vi "SetUnit.vi"(8 "error in":errorcluster, 10 "Unit":T1, 11 "Measure in":refnum<class "Measure.lvclass">) -> (0 "error out":errorcluster, 3 "Measure out":refnum<class "Measure.lvclass">)   [LabVIEW 2021, in "ProligentXMLGenerator.lvlib" / "Measure.lvclass"]
doc: "Defines the name of the unit of the measure value (Ex: kilometer). When a unit symbol is provided, the unit name becomes required.\nDefines the symbol of the unit for the measure value (ex: km). When a unit name is provided, the unit symbol becomes required.\n\nUnit Name vaule is restricted to 30 characters and Unit Symbol is restricted to 20 characters."
uses:
  Measure.lvclass
  Measure.lvclass/Measure.ctl
  Base/Attribute/Attribute.lvclass
  Base/NonEmptyString_20/NonEmptyString_20.lvclass
  Base/NonEmptyString_30/NonEmptyString_30.lvclass
  C:/Projects/proligent-xml-generator-labview/src/ProligentXMLGenerator/Base/NonEmptyString/NonEmptyString.lvclass
  C:/Projects/proligent-xml-generator-labview/src/ProligentXMLGenerator/Base/String/String.lvclass
  C:/Projects/proligent-xml-generator-labview/src/ProligentXMLGenerator/Base/Attribute/Attribute.lvclass
  C:/Projects/proligent-xml-generator-labview/src/ProligentXMLGenerator/Base/NonEmptyString_30/NonEmptyString_30.lvclass
  Unit.ctl
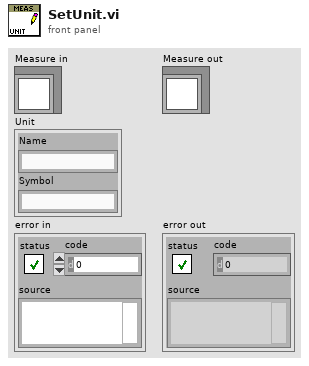
[diagram p1: front panel]
types:
  T1 = typedef "ProligentXMLGenerator.lvlib/Measure.lvclass/Unit.ctl" = cluster{"Name":string, "Symbol":string}
  T2 = typedef "ProligentXMLGenerator.lvlib/Measure.lvclass/Data.ctl" = cluster{"Name":string, "Type":refnum<class "MeasureKind.lvclass">, "Precision":refnum<class "UnsignedByte.lvclass">, "Limit":refnum<class "MeasureLimit.lvclass">, "Characteristics":refnum<class "Characteristic.lvclass">[], "FailureReferences":refnum<class "FailureReference.lvclass">[], "CustomData":refnum<class "CustomData.lvclass">, "MeasureId":refnum<class "Guid.lvclass">, "MeasureTime":refnum<class "DateTime.lvclass">, "Comments":refnum<class "NonNullableString_TruncateAt_255.lvclass">, "Unit":refnum<class "NonEmptyString_30.lvclass">, "Symbol":refnum<class "NonEmptyString_20.lvclass">, "MeasureExecutionStatus":refnum<class "ExecutionStatus.lvclass">}
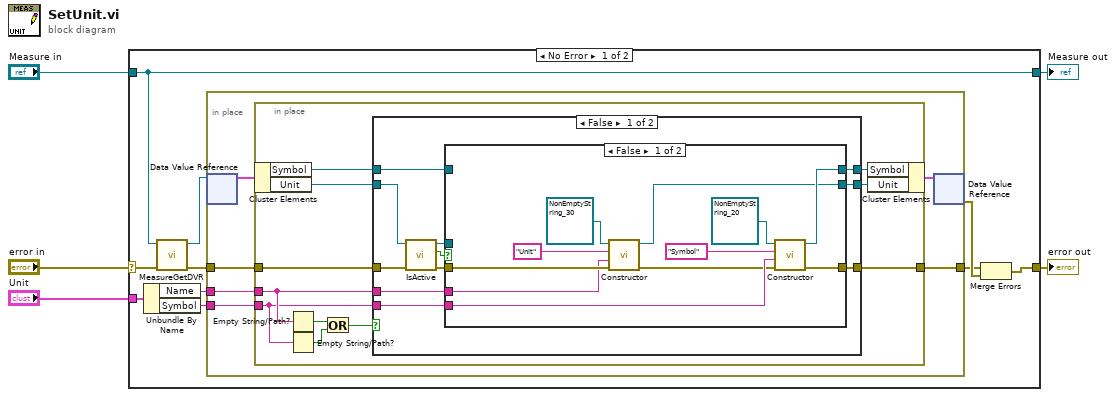
[diagram p0: block diagram]
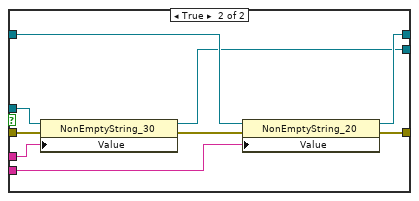
[diagram p2: hidden frame]
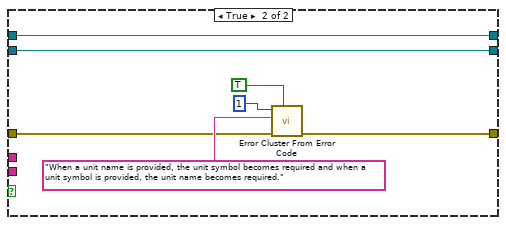
[diagram p3: hidden frame]
diagram:
  n1 = case shown="No Error" "error in" {
    selector: "error in" -> [w13 w71]
    tunnel: "Measure in" -> [w8 w72]
    tunnel: [w10 w71] -> w3
    tunnel: "Unit" -> [w9 _]
    tunnel: [w8 w72] -> w1
    frame No Error {
      n2 = Unbundle By Name(w9) -> ("Name"=w7:string, "Symbol"=w6:string)
      n3 = call "MeasureGetDVR.vi"("error in"=w13, "Measure"=w8) -> ("error out"=w12:errorcluster, "DVRReference"=w14:refnum<data-value>)  [unwired: 8 in]
      n4 = in-place "In Place Element Structure" {
        in-place-border: w12 -> [w21]
        in-place-border: [w20] -> w11
        in-place-border: w7 -> [w19]
        in-place-border: w6 -> [w16]
        n5 = in-place-dvr #1(w14) -> (w18:T2)  [unwired: 1 out]
        n6 = in-place "In Place Element Structure" {
          in-place-border: w21 -> [w25]
          in-place-border: [w32] -> w20
          in-place-border: w19 -> [w24]
          in-place-border: w16 -> [w23]
          n7 = in-place-cluster #2(w18) -> ("Symbol"=w31:refnum<class "NonEmptyString_20.lvclass">, "Unit"=w26:refnum<class "NonEmptyString_30.lvclass">)
          n8 = Empty String/Path?(string/path=w24) -> (empty?=w29:bool)
          n9 = Empty String/Path?(string/path=w23) -> (empty?=w28:bool)
          n10 = Or(x=w29, y=w28) -> (x .or. y?=w22:bool)
          n11 = case shown="False" w22 {
            tunnel: [w43 w68] -> w32
            tunnel: w31 -> [w42 w67]
            tunnel: [w41 w67] -> w30
            tunnel: [w40 w66] -> w27
            tunnel: w26 -> [w39 w66]
            tunnel: w25 -> [w38 w64]
            tunnel: w24 -> [w34 _]
            tunnel: w23 -> [w33 _]
            frame False {
              n12 = call "IsActive.vi"("error in"=w38, "Attribute in"=w39) -> ("error out"=w37:errorcluster, "IsActive"=w36:bool, "Attribute in"=w35:refnum<class "NonEmptyString_30.lvclass">)  [unwired: 7 in]
              n13 = case shown="False" w36 {
                tunnel: w37 -> [w47 w56]
                tunnel: [w52 w63] -> w43
                tunnel: w42 -> [_ w62]
                tunnel: [w54 w61] -> w41
                tunnel: [w45 w60] -> w40
                tunnel: w35 -> [_ w59]
                tunnel: w34 -> [w44 w58]
                tunnel: w33 -> [w53 w57]
                frame False {
                  n14 = call-dynamic "Constructor.vi"("error in"=w47, "Value"=w44, "Name"="Unit", "String in"=refnum<class "NonEmptyString_30.lvclass"> refnum ("ProligentResultProcessor:NonEmptyString_30")) -> ("error out"=w46:errorcluster, "String out"=w45:refnum<class "NonEmptyString_30.lvclass">)  [unwired: 6 in]
                  n15 = call-dynamic "Constructor.vi"("error in"=w46, "Value"=w53, "Name"="Symbol", "String in"=refnum<class "NonEmptyString_20.lvclass"> refnum ("ProligentResultProcessor:NonEmptyString_20")) -> ("error out"=w52:errorcluster, "String out"=w54:refnum<class "NonEmptyString_20.lvclass">)  [unwired: 6 in]
                }
                frame True {
                  n16 = property on="Property Node" class="NonEmptyString_30"(reference=w59, error in=w56, "Value"=w58) -> (reference out=w60:refnum<class "NonEmptyString_30.lvclass">, error out=w55:errorcluster)
                  n17 = property on="Property Node" class="NonEmptyString_20"(reference=w62, error in=w55, "Value"=w57) -> (reference out=w61:refnum<class "NonEmptyString_20.lvclass">, error out=w63:errorcluster)
                }
              }
            }
            frame True {
              n18 = call <vilib>:"Error Cluster From Error Code.vi"("show call chain? (False)"=TRUE, "error in (no error)"=w64, "error message (\"\")"="When a unit name is provided, the unit symbol becomes required and when a unit symbol is provided, the unit name becomes required.", "error code (0)"=1) -> ("error out"=w68:errorcluster)  [unwired: 5 in]
            }
          }
          n19 = in-place-cluster #2("Symbol"=w30, "Unit"=w27) -> (w17:T2)
        }
        n20 = in-place-dvr #1(w17) -> (w15:errorcluster)  [unwired: 1 out]
      }
      n21 = Merge Errors(w11, w15) -> (w10:errorcluster)
    }
    frame Error {
    }
  }
  "error out" <- w3
  "Measure out" <- w1
